vi "getSubPanelScriptEvent.vi"(8 "error in (no error)":errorcluster, 11 "ActionEditor in":refnum<class "ActionEditor.lvclass">) -> (0 "error out":errorcluster, 1 "editing":bool, 2 "ScriptEvent":refnum<class "ScriptEvent.lvclass">, 3 "ActionEditor out":refnum<class "ActionEditor.lvclass">)   [LabVIEW 2011, in "Views.lvlib" / "ScriptEditor.lvlib" / "ActionEditor.lvclass"]
uses:
  ActionEditor.lvclass
  Tools/Scripting/ScriptingEvent/ScriptEvent.lvclass
  ActionEditor.lvclass/ActionEditor.ctl
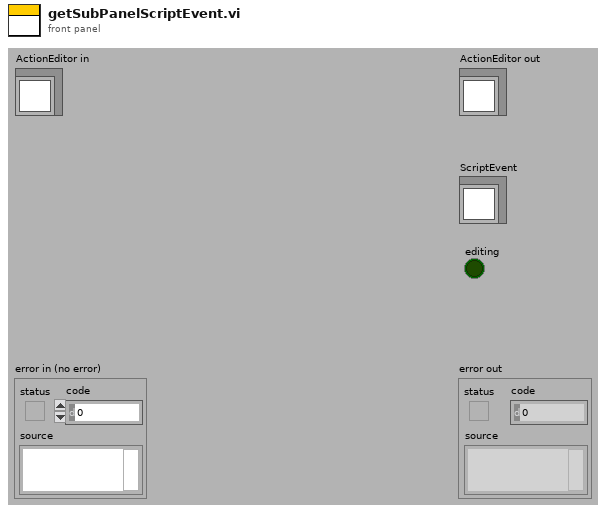
[diagram p1: front panel]
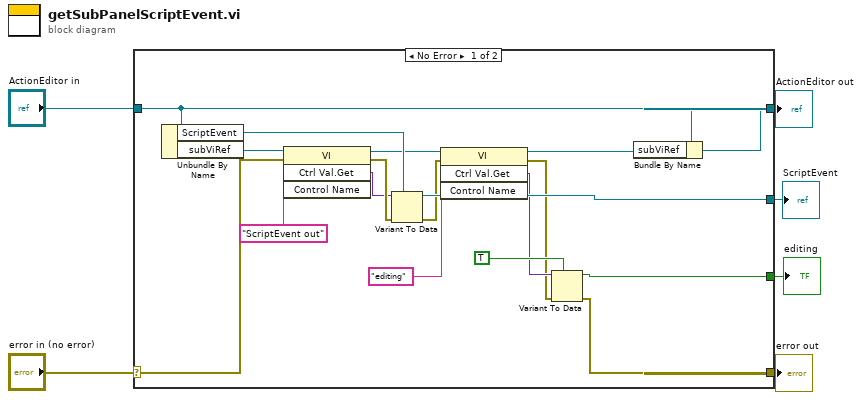
[diagram p0: block diagram]
diagram:
  n1 = case shown="No Error" "error in (no error)" {
    selector: "error in (no error)" -> [w20 w26]
    tunnel: [w8 w26] -> w5
    tunnel: [w16 w25] -> w3
    tunnel: "ActionEditor in" -> [w17 w25]
    tunnel: [w18 _] -> w2
    tunnel: [w9 _] -> w1
    frame No Error {
      n2 = Unbundle By Name(w17) -> ("ScriptEvent"=w19:refnum<class "ScriptEvent.lvclass">, "subViRef"=w21:refnum<vi>)
      n3 = invoke class="VI" method="Ctrl Val.Get"(reference=w21, error in=w20, "Control Name"="ScriptEvent out") -> (reference out=w15:refnum<vi>, error out=w23:errorcluster, "Get Control Value Variant"=w22:variant)  [unwired: 1 in, 1 out]
      n4 = Variant To Data(error in=w23, type=w19, Variant=w22) -> (data=w18:refnum<class "ScriptEvent.lvclass">, error out=w14:errorcluster)
      n5 = invoke class="VI" method="Ctrl Val.Get"(reference=w15, error in=w14, "Control Name"="editing") -> (reference out=w7:refnum<vi>, error out=w10:errorcluster, "Get Control Value Variant"=w11:variant)  [unwired: 1 in, 1 out]
      n6 = Variant To Data(error in=w10, type=TRUE, Variant=w11) -> (data=w9:bool, error out=w8:errorcluster)
      n7 = Bundle By Name(cluster=w17, "subViRef"=w7) -> (w16:refnum<class "ActionEditor.lvclass">)
    }
    frame Error {
    }
  }
  "error out" <- w5
  "ActionEditor out" <- w3
  "ScriptEvent" <- w2
  "editing" <- w1
